vi "Team Processor.vi"(8 "error in (no error)":errorcluster, 10 "Team Count":i32, 11 "Maze 2.0.lvclass":refnum<class "Maze 2.0.lvclass">) -> (0 "error out":errorcluster)   [LabVIEW 2014, in "Maze 2.0.lvclass"]
uses:
  Maze 2.0.lvclass
  Maze 2.0.lvclass/Maze 2.0.ctl
  Runner Cluster.ctl
  Runner/Runner.lvclass
  Move State Cluster.ctl
  Action Enum.ctl
  Direction Enum.ctl
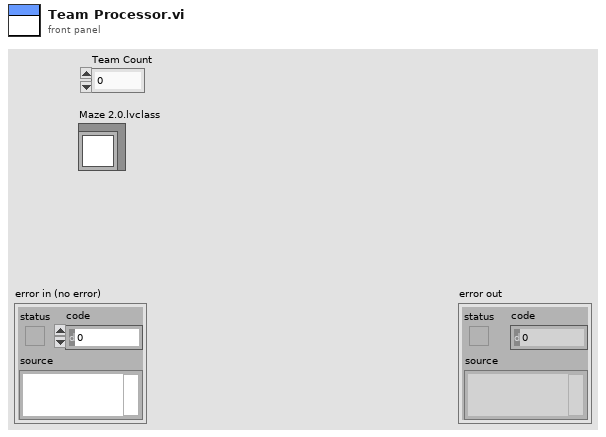
[diagram p1: front panel]
types:
  T1 = typedef "Maze 2.0.lvclass/Move State Cluster.ctl" = cluster{"InPlayPos Dict":variant}
  T2 = typedef "Maze 2.0.lvclass/Runner Cluster.ctl" = cluster{"Alive?":bool, "RunnerRef":refnum<data-value>, "TeamIdx":i32, "Player #":i32, "NextPlay":u32}
  T3 = typedef "Maze 2.0.lvclass/Direction Enum.ctl" = enum16{"NW", "N", "NE", "E", "SE", "S", "SW", "W"}
  T4 = typedef "Maze 2.0.lvclass/Action Enum.ctl" = enum16{"Wait", "Move", "Attack", "Replicate"}
  T5 = cluster{string, "RunnerRef":refnum<data-value>, "Action":T4, "Direction":T3, "Player #":i32, "Replicated":refnum<class "Runner.lvclass">}
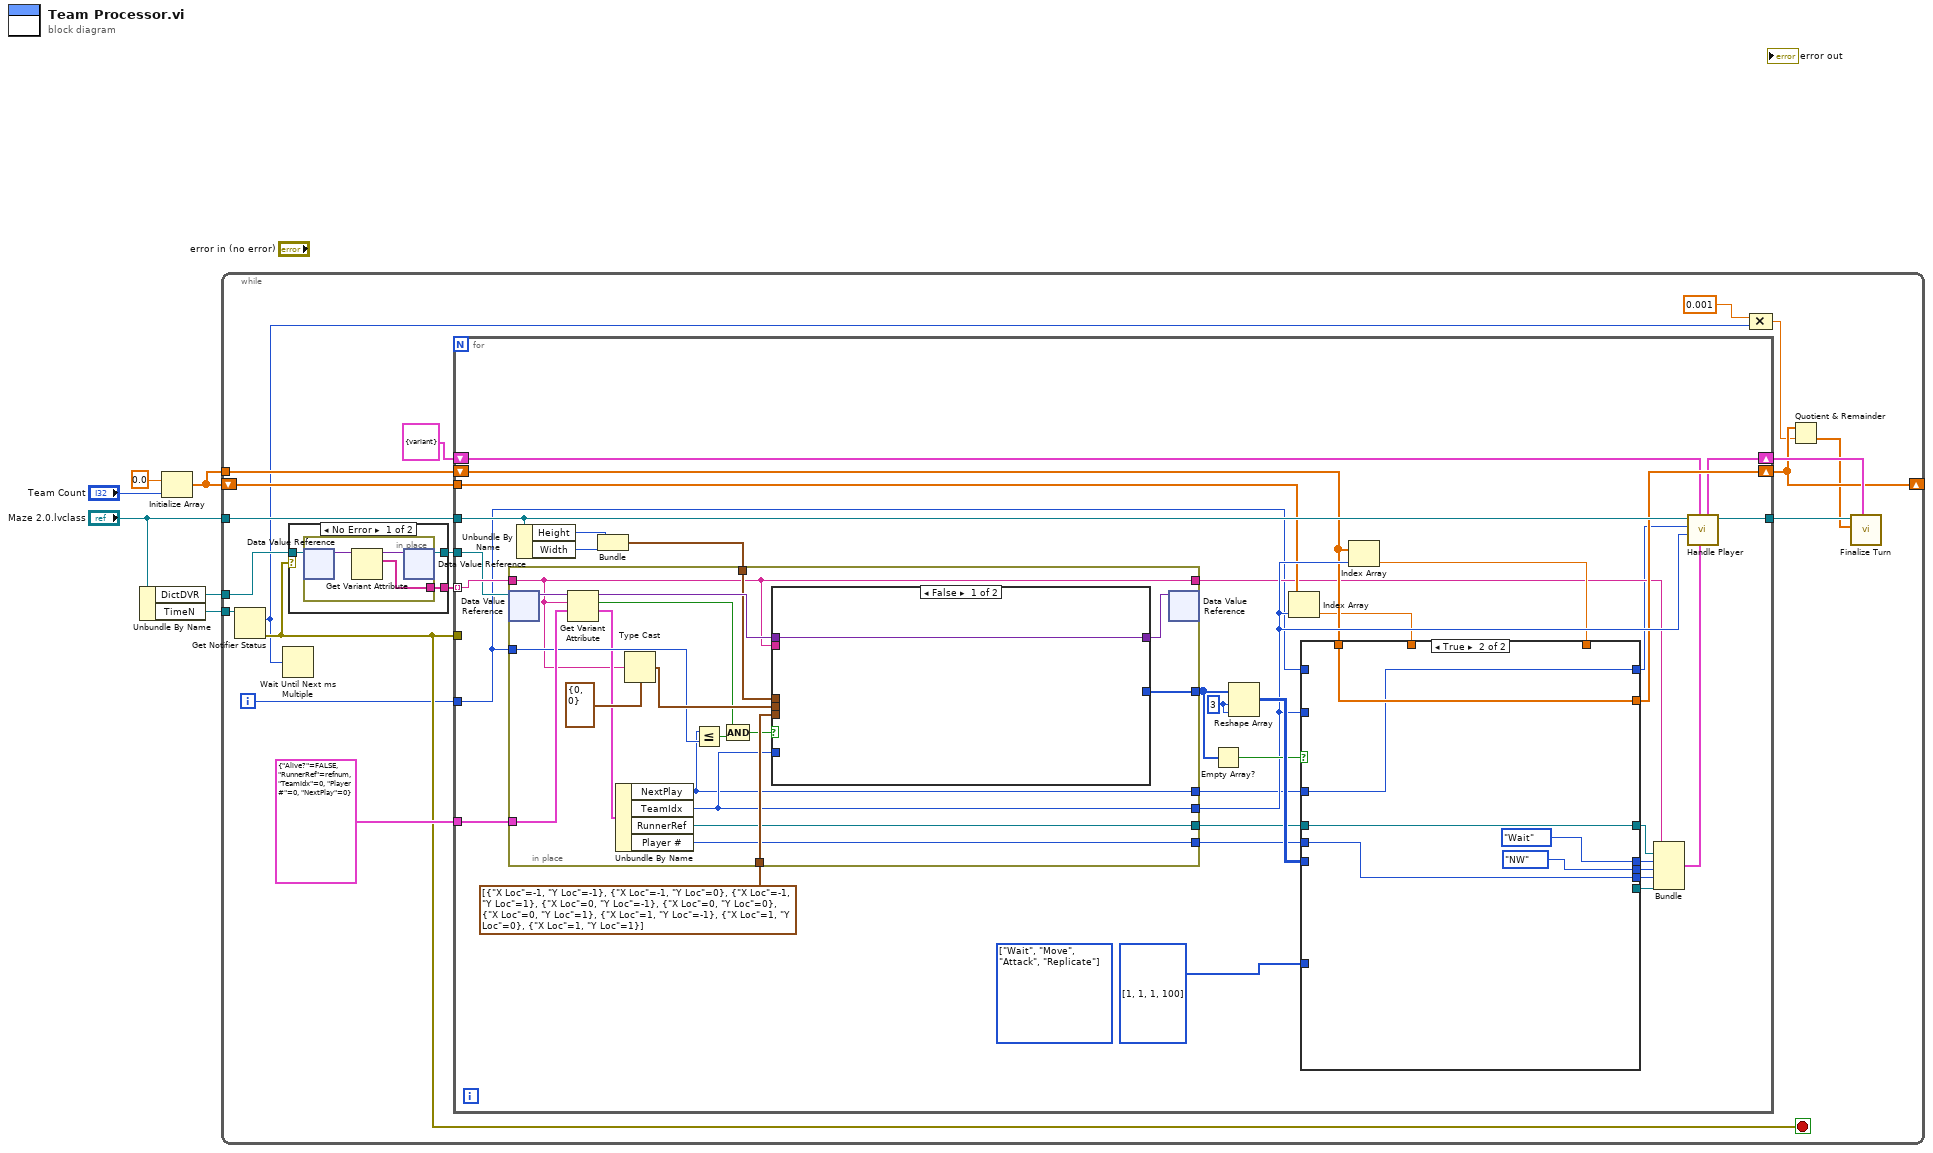
[diagram p0: block diagram]
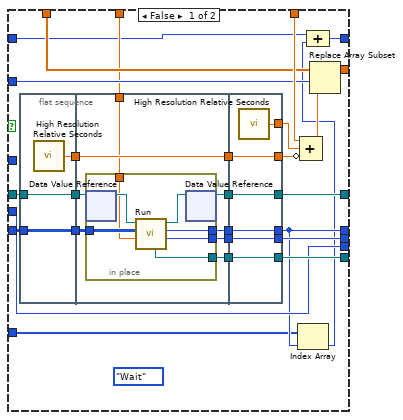
[diagram p3: hidden frame]
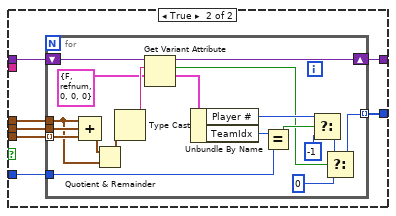
[diagram p4: hidden frame]
diagram:
  n1 = Unbundle By Name("Maze 2.0.lvclass") -> ("DictDVR"=w6:refnum<data-value>, "TimeN"=w5:refnum<notifier>)
  n2 = Initialize Array(0.0, "Team Count") -> (w1:dbl[])
  n3 = while {
    tunnel: w6 -> [w23]
    tunnel: w5 -> [w19]
    tunnel: "Maze 2.0.lvclass" -> [w24]
    shift-right: [w9] -> _
    shift-left: w1 -> [w15]
    tunnel: w1 -> [w16]
    i -> [w17]
    stop <- w18 stop-if-true
    n4 = Get Notifier Status(notifier=w19) -> (current notification=w11:u32, error out=w18:errorcluster)  [unwired: 1 in, 3 out]
    n5 = Wait Until Next ms Multiple(millisecond multiple=w11) -> ()  [unwired: 1 out]
    n6 = case shown="No Error" w18 {
      tunnel: w23 -> [w27 w31]
      tunnel: [w26 _] -> w22
      tunnel: [w25 w31] -> w21
      frame No Error {
        n7 = in-place {
          in-place-border: [w28] -> w26
          n8 = in-place-dvr #1(w27) -> (w30:variant)  [unwired: 1 out]
          n9 = Get Variant Attribute(Variant=w30) -> (duplicate Variant=w29:variant, names=w28:string[])  [unwired: 3 in, 2 out]
          n10 = in-place-dvr #1(w29) -> (w25:refnum<data-value>)  [unwired: 1 out]
        }
      }
      frame Error {
      }
    }
    n11 = for {
      tunnel: w17 -> [w35]
      tunnel: w18 -> [_]
      tunnel: w24 -> [w65]
      tunnel: w22 -> [w64] mode=indexing
      tunnel: w21 -> [w53]
      tunnel: T2 {"Alive?"=FALSE, "RunnerRef"=refnum, "TeamIdx"=0, "Player #"=0, "NextPlay"=0} ("Cluster") -> [w63]
      shift-right: [w49] -> w9
      shift-left: w16 -> [w51]
      tunnel: w15 -> [w50]
      shift-right: [w47] -> w13
      shift-left: T1 {"InPlayPos Dict"=variant(i32[] [])} ("Cluster") -> [w48]
      tunnel: [w46] -> w12
      (unwired) T4[] [enum."Wait", enum."Move", enum."Attack", enum."Replicate"] items=["Wait", "Move", "Attack", "Replicate"]
      w60 = 3 ("dimension size")
      n12 = Unbundle By Name(w65) -> ("Height"=w59:i32, "Width"=w58:i32)
      n13 = Bundle("Height"=w59, "Width"=w58) -> (w57:cluster{"Height":i32, "Width":i32})  [unwired: 1 in]
      n14 = in-place {
        in-place-border: cluster{"X Loc":i32, "Y Loc":i32}[] [{"X Loc"=-1, "Y Loc"=-1}, {"X Loc"=-1, "Y Loc"=0}, {"X Loc"=-1, "Y Loc"=1}, {"X Loc"=0, "Y Loc"=-1}, {"X Loc"=0, "Y Loc"=0}, {"X Loc"=0, "Y Loc"=1}, {"X Loc"=1, "Y Loc"=-1}, {"X Loc"=1, "Y Loc"=0}, {"X Loc"=1, "Y Loc"=1}] -> [w141]
        in-place-border: [w140] -> w56
        in-place-border: w64 -> [w127]
        in-place-border: w63 -> [w138]
        in-place-border: w35 -> [w135]
        in-place-border: w57 -> [w131]
        in-place-border: [w128] -> w54
        in-place-border: [w127] -> w39
        in-place-border: [w125] -> w52
        in-place-border: [w124] -> w37
        in-place-border: [w123] -> w32
        n15 = in-place-dvr #2(w53) -> (w139:variant)  [unwired: 1 out]
        n16 = Get Variant Attribute(Variant=w139, name=w127, default value (empty Variant)=w138) -> (duplicate Variant=w134:variant, found=w130:bool, value=w129:T2)  [unwired: 1 in, 1 out]
        n17 = Unbundle By Name(w129) -> ("NextPlay"=w123:u32, "TeamIdx"=w125:i32, "RunnerRef"=w128:refnum<data-value>, "Player #"=w124:i32)
        n18 = Type Cast(type=cluster{"Y":i32, "X":i32} {"Y"=0, "X"=0}, x=w127) -> (*(type *) &x=w136:cluster{"Y":i32, "X":i32})
        n19 = Less Or Equal?(x=w123, y=w135) -> (x <= y?=w133:bool)
        n20 = Compound Arithmetic op=AND(w130, w133) -> (w126:bool)
        n21 = case shown="False" w126 {
          tunnel: w141 -> [_ w149]
          tunnel: [_ w148] -> w140
          tunnel: w125 -> [_ w147]
          tunnel: w136 -> [_ w146]
          tunnel: w134 -> [w142 w145]
          tunnel: [w142 w144] -> w132
          tunnel: w131 -> [_ w143]
          tunnel: w127 -> [_ _]
          frame False {
          }
          frame True {
            n22 = for {
              tunnel: w146 -> [w168]
              tunnel: w143 -> [w165]
              tunnel: w149 -> [w167] mode=indexing
              tunnel: [w163] -> w148 mode=indexing
              tunnel: w147 -> [w157]
              shift-right: [w150] -> w144
              shift-left: w145 -> [w155]
              n23 = Compound Arithmetic op=ADD(w165, w168, w167) -> (w166:cluster{i32, i32})
              n24 = Quotient & Remainder(x=w166, y=w165) -> (x-y*floor(x/y)=w156:cluster{i32, i32})  [unwired: 1 out]
              n25 = Type Cast(x=w156) -> (*(type *) &x=w154:string)  [unwired: 1 in]
              n26 = Get Variant Attribute(Variant=w155, name=w154, default value (empty Variant)=T2 {"Alive?"=FALSE, "RunnerRef"=refnum, "TeamIdx"=0, "Player #"=0, "NextPlay"=0} ("Cluster")) -> (duplicate Variant=w150:variant, found=w151:bool, value=w152:T2)  [unwired: 1 in, 1 out]
              n27 = Unbundle By Name(w152) -> ("Player #"=w161:i32, "TeamIdx"=w159:i32)
              n28 = Equal?(x=w159, y=w157) -> (x = y?=w158:bool)
              n29 = Select(t=w161, s=w158, f=-1) -> (s? t:f=w162:i32)
              n30 = Select(t=w162, s=w151, f=0) -> (s? t:f=w163:i32)
            }
          }
        }
        n31 = in-place-dvr #2(w132) -> ()  [unwired: 2 out]
      }
      n32 = Empty Array?(array=w56) -> (empty?=w55:bool)
      n33 = Reshape Array(w56, w60, w60) -> (w61:i32[][])
      n34 = Index Array(array=w50, index=w52) -> (element=w40:dbl)
      n35 = Index Array(array=w51, index=w52) -> (element=w45:dbl)
      n36 = case shown="True" w55 {
        tunnel: w54 -> [w85 w119]
        tunnel: w61 -> [w84 _]
        tunnel: w45 -> [w81 _]
        tunnel: w51 -> [w80 w122]
        tunnel: [w78 w122] -> w49
        tunnel: [w68 Action_Enum."Wait" ("Action")] -> w44
        tunnel: [w77 Direction_Enum."NW" ("Direction")] -> w43
        tunnel: [w76 _] -> w42
        tunnel: w52 -> [w75 _]
        tunnel: w40 -> [w74 _]
        tunnel: [w73 w119] -> w38
        tunnel: w37 -> [w71 w118]
        tunnel: [w71 w118] -> w36
        tunnel: w35 -> [w70 _]
        tunnel: [w69 w117] -> w34
        tunnel: u32[] [1, 1, 1, 100] -> [w67 _]
        tunnel: w32 -> [_ w117]
        frame False {
          (unwired) Action_Enum."Wait" ("Action")
          n37 = flat-sequence {
            tunnel: w84 -> [w94]
            tunnel: w85 -> [w95]
            tunnel: [w95] -> w92
            tunnel: [w94] -> w91
            tunnel: [w93] -> w90
            tunnel: [w101] -> w89
            tunnel: [w100] -> w88
            tunnel: [w99] -> w87
            tunnel: w92 -> [w103]
            tunnel: w91 -> [w102]
            tunnel: w90 -> [w98]
            tunnel: [w98] -> w86
            tunnel: w74 -> [w97]
            tunnel: [w96] -> w72
            tunnel: [w114] -> w76
            tunnel: [w115] -> w77
            tunnel: [w116] -> w68
            tunnel: w89 -> [w116]
            tunnel: w88 -> [w115]
            tunnel: w87 -> [w114]
            tunnel: [w113] -> w82
            tunnel: w86 -> [w113]
            tunnel: [w112] -> w83
            tunnel: [w111] -> w73
            tunnel: w72 -> [w111]
            frame #0 {
              n38 = call <vilib>:"High Resolution Relative Seconds.vi"() -> ("relative seconds"=w93:dbl)
            }
            frame #1 {
              n39 = in-place {
                in-place-border: w102 -> [w108]
                in-place-border: [w107] -> w101
                in-place-border: [w106] -> w100
                in-place-border: [w105] -> w99
                in-place-border: w97 -> [w104]
                n40 = in-place-dvr #3(w103) -> (w110:refnum<class "Runner.lvclass">)  [unwired: 1 out]
                n41 = call-dynamic "Run.vi"("s on last turn"=w104, "Maze (0: Empty, -1: Enemy. >0: Teammate"=w108, "Runner in"=w110) -> ("Direction"=w106:T3, "Action"=w107:T4, "Runner out"=w109:refnum<class "Runner.lvclass">, "Replicated"=w105:refnum<class "Runner.lvclass">)  [unwired: 4 in, 1 out]
                n42 = in-place-dvr #3(w109) -> (w96:refnum<data-value>)  [unwired: 1 out]
              }
            }
            frame #2 {
              n43 = call <vilib>:"High Resolution Relative Seconds.vi"() -> ("relative seconds"=w112:dbl)
            }
          }
          n44 = Index Array(array=w67, index=w68) -> (element=w66:u32)
          n45 = Compound Arithmetic op=ADD(w81, w83, invert w82) -> (w79:dbl)
          n46 = Compound Arithmetic op=ADD(w70, w66) -> (w69:u32)
          n47 = Replace Array Subset(array=w80, new element=w79, index=w75) -> (w78:dbl[])
        }
        frame True {
        }
      }
      n48 = Bundle(w39, "RunnerRef"=w38, "Action"=w44, "Direction"=w43, "Player #"=w36, "Replicated"=w42) -> (w41:T5)  [unwired: 1 in]
      n49 = call "Handle Player.vi"("Move"=w41, "Move in"=w48, "Team"=w52, "Turn"=w34, "Maze 2.0 in"=w65) -> ("Maze 2.0 out"=w46:refnum<class "Maze 2.0.lvclass">, "Move out"=w47:T1)  [unwired: 4 in, 1 out]
    }
    n50 = Compound Arithmetic op=MULTIPLY(0.001, w11) -> (w8:dbl)
    n51 = Quotient & Remainder(x=w9, y=w8) -> (floor(x/y)=w7:dbl[])  [unwired: 1 out]
    n52 = call "Finalize Turn.vi"("Move State"=w13, "Turn Penalty[team]"=w7, "Maze 2.0 in"=w12) -> ()  [unwired: 7 in, 2 out]
  }
